vi "Generate Display Data.vi"(5 "Cal Runtime Cfg":T4, 7 "Config Data":T3(array[cluster]), 8 "error in":errorcluster, 10 "CorrOffset File In":T6, 11 "Site Data":T1[](array[typedef])) -> (0 "error out":errorcluster, 1 "Data String":string[][](array[string]), 2 "Col Header String":string[](array[string]), 3 "Limit Status":T5, 6 "Final Offset":T7)   [LabVIEW 2020, in "GUCalibration2.lvlib"]
uses:
  GUCalibration2.lvlib
  Controls/Config Data Type.ctl
  Controls/Site Data Element.ctl
  Controls/Site Raw Data Element.ctl
  <vilib>/Analysis/baseanly.llb/Mean (DBL).vi
  <vilib>/Analysis/NI_AALBase.lvlib
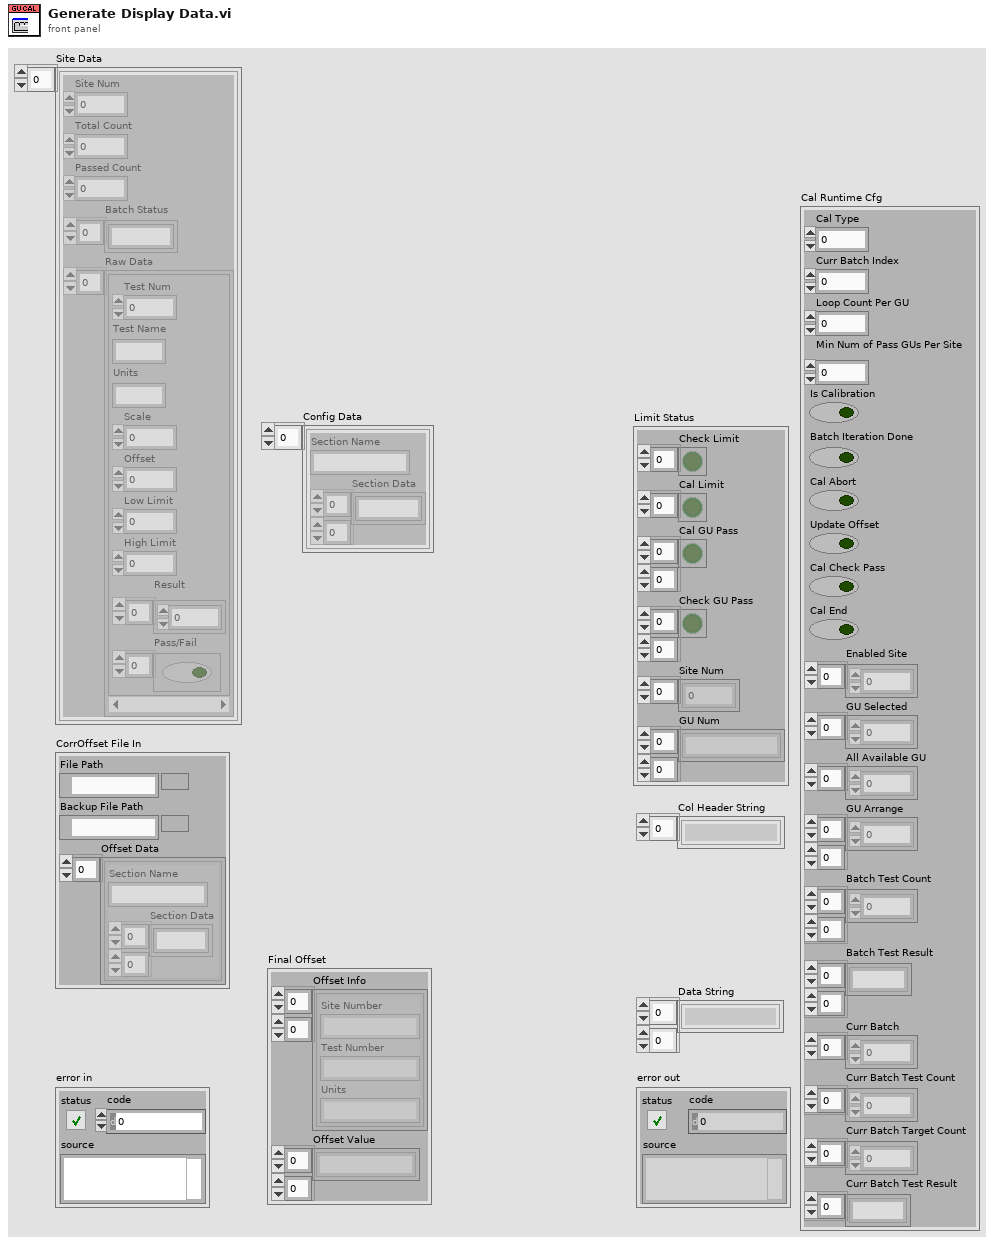
[diagram p1: front panel]
types:
  T1 = typedef "GUCalibration2.lvlib/Site Data Element.ctl" = cluster{"Site Num":i32, "Total Count":i32, "Passed Count":i32, "Batch Status":string[], "Raw Data":T2[]}
  T2 = typedef "GUCalibration2.lvlib/Site Raw Data Element.ctl" = cluster{"Test Num":u32, "Test Name":string, "Units":string, "Scale":i8, "Offset":dbl, "Low Limit":dbl, "High Limit":dbl, "Result":dbl[], "Pass/Fail":bool[]}
  T3 = cluster{"Section Name":string, "Section Data":string[][]}[]
  T4 = typedef "GUCalibration2.lvlib/Config Data Type.ctl" = cluster{"Cal Type":i32, "Curr Batch Index":i32, "Loop Count Per GU":i32, "Min Num of Pass GUs Per Site":i32, "Is Calibration":bool, "Batch Iteration Done":bool, "Cal Abort":bool, "Update Offset":bool, "Cal Check Pass":bool, "Cal End":bool, "Enabled Site":i32[], "GU Selected":i32[], "All Available GU":i32[], "GU Arrange":i32[][], "Batch Test Count":i32[][], "Batch Test Result":string[][], "Curr Batch":i32[], "Curr Batch Test Count":i32[], "Curr Batch Target Count":i32[], "Curr Batch Test Result":string[]}
  T5 = cluster{"Check Limit":bool[], "Cal Limit":bool[], "Cal GU Pass":bool[][], "Check GU Pass":bool[][], "Site Num":i32[], "GU Num":string[][]}
  T6 = cluster{"File Path":path, "Backup File Path":path, "Offset Data":cluster{"Section Name":string, "Section Data":string[][]}[]}
  T7 = cluster{"Offset Info":cluster{"Site Number":string, "Test Number":string, "Units":string}[][], "Offset Value":string[][]}
  T8 = cluster{string, "String":string, "Combined Units":string}
  T9 = cluster{cluster{string, "String":string, "Combined Units":string}[][], string[][]}
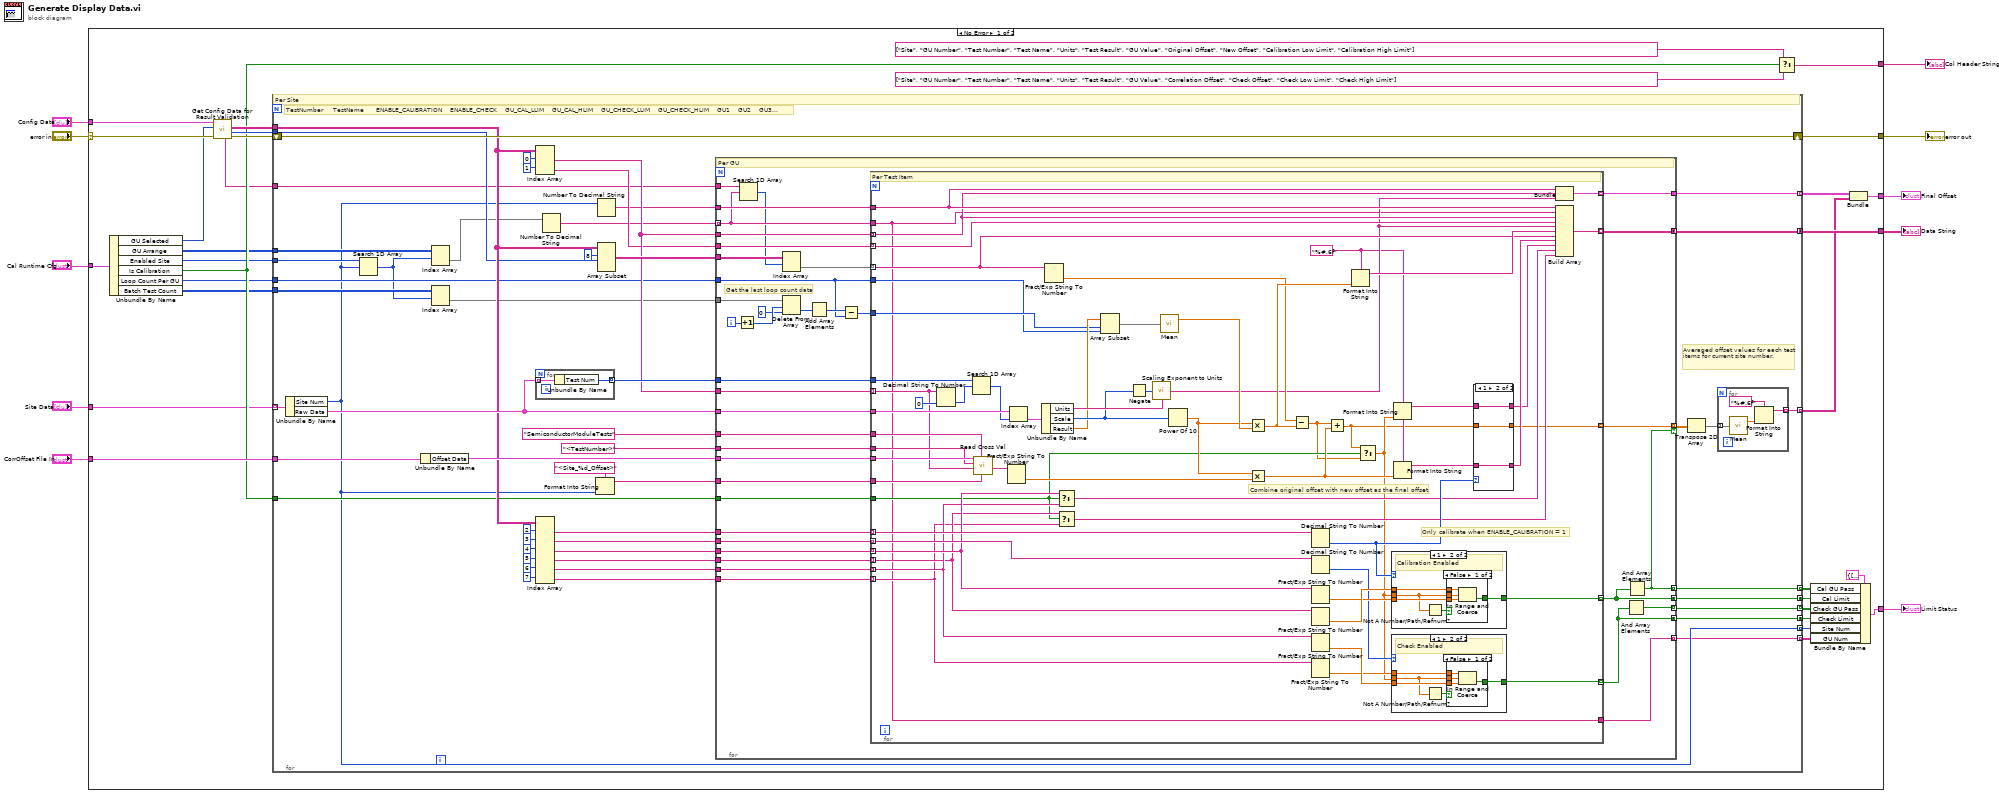
[diagram p0: block diagram]
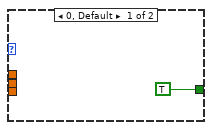
[diagram p2: hidden frame]
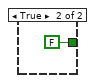
[diagram p3: hidden frame]
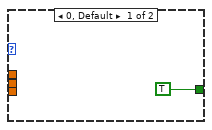
[diagram p4: hidden frame]
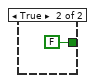
[diagram p5: hidden frame]
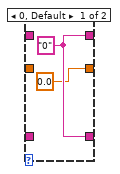
[diagram p6: hidden frame]
diagram:
  n1 = case shown="No Error" "error in" {
    selector: "error in" -> [w39 w225]
    tunnel: [w41 w225] -> w10
    tunnel: [w30 _] -> w8
    tunnel: "CorrOffset File In" -> [w40 _]
    tunnel: [w35 _] -> w7
    tunnel: [w32 _] -> w6
    tunnel: [w26 _] -> w1
    tunnel: "Cal Runtime Cfg" -> [w25 _]
    tunnel: "Config Data" -> [w17 _]
    tunnel: "Site Data" -> [w16 _]
    frame No Error {
      n2 = Unbundle By Name(w25) -> ("GU Selected"=w22:i32[], "GU Arrange"=w21:i32[][], "Enabled Site"=w20:i32[], "Is Calibration"=w24:bool, "Loop Count Per GU"=w23:i32, "Batch Test Count"=w18:i32[][])
      n3 = call "Get Config Data for Result Validation.vi"("error in"=w39, "GU Selected"=w22, "Config Data"=w17) -> ("error out"=w38:errorcluster, "Number of GU"=w36:i32, "Config Data"=w37:string[][], "GU Numbers"=w19:string[])  [unwired: 4 in, 1 out]
      n4 = for {
        shift-right: [w81] -> w41
        shift-left: w38 -> [w81]
        tunnel: w16 -> [w93] mode=indexing
        tunnel: w40 -> [w89]
        tunnel: [w82] -> w27 mode=concatenating
        tunnel: [w83] -> w28 mode=concatenating
        tunnel: w37 -> [w80]
        tunnel: w36 -> [w79]
        tunnel: w23 -> [w73]
        tunnel: [w60] -> w35 mode=concatenating
        tunnel: [w57] -> w33 mode=indexing
        tunnel: [w55] -> w34 mode=indexing
        tunnel: w24 -> [w54]
        tunnel: w21 -> [w52]
        tunnel: w20 -> [w53]
        tunnel: w19 -> [w49]
        tunnel: w18 -> [w48]
        tunnel: [w45] -> w15 mode=indexing
        tunnel: [w44] -> w14 mode=indexing
        tunnel: [w43] -> w13 mode=indexing
        tunnel: [w42] -> w11 mode=indexing
        # "Averaged offset values for each test items for current site number."
        # "TestNumber     TestName      ENABLE_CALIBRATION    ENABLE_CHECK    GU_CAL_LLIM    GU_CAL_HLIM    GU_CHECK_LLIM    GU_CHECK_HLIM    GU1    GU2    GU3..."
        # "Per Site"
        n5 = Unbundle By Name(w93) -> ("Site Num"=w43:i32, "Raw Data"=w90:T2[])
        n6 = Search 1D Array(1D array=w53, element=w43) -> (index of element=w46:i32)  [unwired: 1 in]
        n7 = Unbundle By Name(w89) -> ("Offset Data"=w88:T3)
        n8 = Index Array(array=w52, index (row)=w46) -> (element=w51:i32[])  [unwired: 1 in]
        n9 = Index Array(array=w48, index (row)=w46) -> (element=w47:i32[])  [unwired: 1 in]
        n10 = Index Array(array=w80, index (row) #1=0 ("index (row)"), index (row) #2=1 ("index (row)")) -> (element #1=w76:string[], element #2=w74:string[])  [unwired: 2 in]
        n11 = for {
          tunnel: w90 -> [w224] mode=indexing
          tunnel: [w223] -> w91 mode=indexing
          n12 = Unbundle By Name(w224) -> ("Test Num"=w223:u32)
        }
        n13 = Index Array(array=w80, index (row) #1=2 ("index (row)"), index (row) #2=3 ("index (row)"), index (row) #3=4 ("index (row)"), index (row) #4=5 ("index (row)"), index (row) #5=6 ("index (row)"), index (row) #6=7 ("index (row)")) -> (element #1=w61:string[], element #2=w62:string[], element #3=w63:string[], element #4=w64:string[], element #5=w65:string[], element #6=w66:string[])  [unwired: 6 in]
        n14 = Number To Decimal String(number=w51) -> (decimal integer string=w50:string[])  [unwired: 1 in]
        n15 = Format Into String(format string="<Site_%d_Offset>", w43) -> (resulting string=w85:string)  [unwired: 2 in, 1 out]
        n16 = Number To Decimal String(number=w43) -> (decimal integer string=w56:string)  [unwired: 1 in]
        n17 = Array Subset(array=w80, index (row)=8 ("index"), length (row)=w79) -> (w77:string[][])  [unwired: 2 in]
        n18 = for {
          tunnel: w76 -> [w135]
          tunnel: w91 -> [w134]
          tunnel: w90 -> [w133]
          tunnel: w88 -> [w132]
          tunnel: "<TestNumber>" ("Col Header Name") -> [w131]
          tunnel: w85 -> [w130]
          tunnel: "SemiconductorModuleTests" ("Section Name") -> [w129]
          tunnel: w62 -> [w128]
          tunnel: w63 -> [w127]
          tunnel: w64 -> [w126]
          tunnel: w65 -> [w125]
          tunnel: w66 -> [w124]
          tunnel: [w102] -> w83 mode=concatenating
          tunnel: [w100] -> w82 mode=concatenating
          tunnel: w61 -> [w123]
          tunnel: w77 -> [w113]
          tunnel: w56 -> [w122]
          tunnel: w50 -> [w114] mode=indexing
          tunnel: w76 -> [w121]
          tunnel: w74 -> [w120]
          tunnel: w73 -> [w104]
          tunnel: [w119] -> w60 mode=concatenating
          tunnel: [w118] -> w59 mode=indexing if=w101
          tunnel: [w117] -> w55
          tunnel: w54 -> [w116]
          tunnel: w49 -> [w115]
          tunnel: w47 -> [w107]
          tunnel: [w101] -> w45 mode=indexing
          tunnel: [w99] -> w44 mode=indexing
          tunnel: [w98] -> w42 mode=indexing
          i -> [w106]
          # "Get the last loop count data"
          # "Per GU"
          n19 = Increment(x=w106) -> (x+1=w110:i32)
          n20 = Search 1D Array(1D array=w115, element=w114) -> (index of element=w112:i32)  [unwired: 1 in]
          n21 = Index Array(array=w113, index (row)=w112) -> (element=w111:string[])  [unwired: 1 in]
          n22 = Delete From Array(array=w107, length=w110, index=0) -> (deleted portion=w108:i32[])  [unwired: 1 out]
          n23 = Add Array Elements(numeric array=w108) -> (sum=w105:i32)
          n24 = Subtract(x=w105, y=w104) -> (x-y=w103:i32)
          n25 = for {
            tunnel: w135 -> [w173] mode=indexing
            tunnel: w134 -> [w195]
            tunnel: w133 -> [w194]
            tunnel: w132 -> [w193]
            tunnel: w131 -> [w192]
            tunnel: w130 -> [w191]
            tunnel: w129 -> [w190]
            tunnel: w111 -> [w164] mode=indexing
            tunnel: w123 -> [w189] mode=indexing
            tunnel: w128 -> [w177] mode=indexing
            tunnel: w127 -> [w151] mode=indexing
            tunnel: w126 -> [w148] mode=indexing
            tunnel: [w174] -> w102 mode=indexing
            tunnel: w125 -> [w149] mode=indexing
            tunnel: w124 -> [w147] mode=indexing
            tunnel: [w170] -> w100 mode=indexing
            tunnel: w122 -> [w158]
            tunnel: w114 -> [w136]
            tunnel: w121 -> [w157] mode=indexing
            tunnel: w120 -> [w169] mode=indexing
            tunnel: w104 -> [w139]
            tunnel: [w162] -> w119 mode=indexing
            tunnel: [w145] -> w118 mode=indexing
            tunnel: [w156] -> w117 mode=indexing
            tunnel: w116 -> [w143]
            tunnel: w103 -> [w140]
            tunnel: [w136] -> w98
            w144 = "%#.6f" ("format string")
            # "Combine original offset with new offset as the final offset"
            # "Only calibrate when ENABLE_CALIBRATION = 1"
            # "Per Test Item"
            n26 = Decimal String To Number(string=w173, default (0L)=u32 0 ("default (0 I32)")) -> (number=w180:u32)  [unwired: 1 in, 1 out]
            n27 = Search 1D Array(1D array=w195, element=w180) -> (index of element=w181:i32)  [unwired: 1 in]
            n28 = call "Read Cross Val.vi"("Col Header Name 2"=w191, "Section Name"=w190, "Col Header Val 1"=w173, "Col Header Name 1"=w192, "Config Data"=w193) -> ("Col Header Val 2"=w183:string)  [unwired: 3 in, 3 out]
            n29 = Fract/Exp String To Number(string=w183) -> (number=w182:dbl)  [unwired: 3 in, 1 out]
            n30 = Index Array(array=w194, index=w181) -> (element=w187:T2)
            n31 = Unbundle By Name(w187) -> ("Units"=w185:string, "Scale"=w184:i8, "Result"=w168:dbl[])
            n32 = Fract/Exp String To Number(string=w164) -> (number=w160:dbl)  [unwired: 3 in, 1 out]
            n33 = Select(t=w151, s=w143, f=w149) -> (s? t:f=w152:string)
            n34 = Select(t=w148, s=w143, f=w147) -> (s? t:f=w150:string)
            n35 = Array Subset(array=w168, index=w140, length=w139) -> (w138:dbl[])
            n36 = Negate(x=w184) -> (-x=w186:i8)
            n37 = call "Scaling Exponent to Units.vi"("Units"=w185, "Scaling Exponent"=w186) -> ("Combined Units"=w155:string)  [unwired: 2 in]
            n38 = call-poly <vilib>:"Mean.vi"("X"=w138) -> ("mean"=w167:dbl)  [unwired: 1 out]
            n39 = Power Of 10(x=w184) -> (10^x=w166:dbl)
            n40 = Multiply(x=w166, y=w167) -> (x*y=w161:dbl)
            n41 = Multiply(x=w166, y=w182) -> (x*y=w146:dbl)
            n42 = Subtract(x=w160, y=w161) -> (x-y=w142:dbl)
            n43 = Decimal String To Number(string=w189) -> (number=w154:i32)  [unwired: 2 in, 1 out]
            n44 = Decimal String To Number(string=w177) -> (number=w153:i32)  [unwired: 2 in, 1 out]
            n45 = Fract/Exp String To Number(string=w151) -> (number=w175:dbl)  [unwired: 3 in, 1 out]
            n46 = Fract/Exp String To Number(string=w148) -> (number=w176:dbl)  [unwired: 3 in, 1 out]
            n47 = Fract/Exp String To Number(string=w149) -> (number=w172:dbl)  [unwired: 3 in, 1 out]
            n48 = Fract/Exp String To Number(string=w147) -> (number=w171:dbl)  [unwired: 3 in, 1 out]
            n49 = Add(x=w142, y=w146) -> (x+y=w137:dbl)
            n50 = Format Into String(format string=w144, w161) -> (resulting string=w165:string)  [unwired: 2 in, 1 out]
            n51 = Select(t=w137, s=w143, f=w142) -> (s? t:f=w141:dbl)
            n52 = case shown="1" w154 {
              tunnel: w141 -> [_ w209]
              tunnel: w175 -> [_ w212]
              tunnel: w176 -> [_ w211]
              tunnel: [TRUE w210] -> w174
              frame 0, Default {
              }
              frame 1 {
                # "Calibration Enabled"
                n53 = Not A Number/Path/Refnum?(number/path/refnum=w209) -> (NaN/Path/Refnum?=w208:bool)
                n54 = case shown="False" w208 {
                  tunnel: w209 -> [w216 _]
                  tunnel: w212 -> [w215 _]
                  tunnel: w211 -> [w214 _]
                  tunnel: [w213 FALSE] -> w210
                  frame False {
                    n55 = In Range and Coerce(upper limit=w214, x=w216, lower limit=w215) -> (In Range?=w213:bool)  [unwired: 1 out]
                  }
                  frame True {
                  }
                }
              }
            }
            n56 = case shown="1" w153 {
              tunnel: w141 -> [_ w198]
              tunnel: w172 -> [_ w201]
              tunnel: w171 -> [_ w200]
              tunnel: [TRUE w199] -> w170
              frame 0, Default {
              }
              frame 1 {
                # "Check Enabled"
                n57 = Not A Number/Path/Refnum?(number/path/refnum=w198) -> (NaN/Path/Refnum?=w197:bool)
                n58 = case shown="False" w197 {
                  tunnel: w198 -> [w205 _]
                  tunnel: w201 -> [w204 _]
                  tunnel: w200 -> [w203 _]
                  tunnel: [w202 FALSE] -> w199
                  frame False {
                    n59 = In Range and Coerce(upper limit=w203, x=w205, lower limit=w204) -> (In Range?=w202:bool)  [unwired: 1 out]
                  }
                  frame True {
                  }
                }
              }
            }
            n60 = Format Into String(format string=w144, w141) -> (resulting string=w178:string)  [unwired: 2 in, 1 out]
            n61 = Format Into String(format string=w144, w146) -> (resulting string=w179:string)  [unwired: 2 in, 1 out]
            n62 = case shown="1" w154 {
              tunnel: [w219 w222] -> w163
              tunnel: w179 -> [_ w222]
              tunnel: [w219 w221] -> w159
              tunnel: w178 -> [_ w221]
              tunnel: [0.0 w220] -> w145
              tunnel: w137 -> [_ w220]
              frame 0, Default {
                w219 = "0"
              }
              frame 1 {
              }
            }
            n63 = Bundle(w158, "String"=w157, "Combined Units"=w155) -> (w156:T8)  [unwired: 1 in]
            n64 = Build Array(w158, w136, w157, w169, w155, w165, w164, w163, w159, w152, w150) -> (w162:string[])
          }
          n65 = And Array Elements(Boolean array=w100) -> (logical AND=w99:bool)
          n66 = And Array Elements(Boolean array=w102) -> (logical AND=w101:bool)
        }
        n67 = Transpose 2D Array(2D array=w59) -> (transposed array=w58:dbl[][])
        n68 = for {
          tunnel: w58 -> [w97] mode=indexing
          tunnel: [w94] -> w57 mode=indexing
          n69 = call-poly <vilib>:"Mean.vi"("X"=w97) -> ("mean"=w95:dbl)  [unwired: 1 out]
          n70 = Format Into String(format string="%#.6f", w95) -> (resulting string=w94:string)  [unwired: 2 in, 1 out]
        }
      }
      n71 = Select(t=string[] ["Site", "GU Number", "Test Number", "Test Name", "Units", "Test Result", "GU Value", "Original Offset", "New Offset", "Calibration Low Limit", "Calibration High Limit"] ("Column Data"), s=w24, f=string[] ["Site", "GU Number", "Test Number", "Test Name", "Units", "Test Result", "GU Value", "Correlation Offset", "Check Offset", "Check Low Limit", "Check High Limit"] ("Column Data")) -> (s? t:f=w30:string[])
      n72 = Bundle By Name(cluster=T5 {"Check Limit"=[], "Cal Limit"=[], "Cal GU Pass"=[], "Check GU Pass"=[], "Site Num"=[], "GU Num"=[]} ("Limit Status"), "Cal GU Pass"=w15, "Cal Limit"=w28, "Check GU Pass"=w14, "Check Limit"=w27, "Site Num"=w13, "GU Num"=w11) -> (w26:T5)
      n73 = Bundle(w34, w33) -> (w32:T9)  [unwired: 1 in]
    }
    frame Error {
    }
  }
  "error out" <- w10
  "Col Header String" <- w8
  "Data String" <- w7
  "Final Offset" <- w6
  "Limit Status" <- w1
